vi "Destroy.vi"(8 "Error In":errorcluster, 11 "Parser":refnum<class "Parser.lvclass">) -> (0 "Error Out":errorcluster)   [LabVIEW 2017, in "Mustache.lvlib" / "Parser.lvclass"]
uses:
  Parser.lvclass
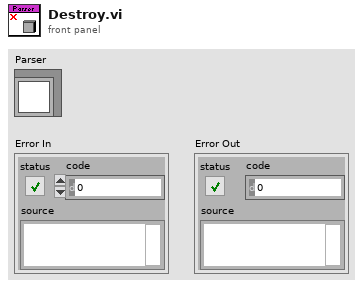
[diagram p1: front panel]
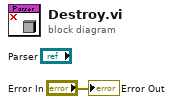
[diagram p0: block diagram]
diagram:
  "Error Out" <- "Error In"
